vi "PicohrdlStreamingRun.vi"(5 "noOfChannels":i16=2, 7 "conversionTime":i16(ring) items=["60 ms", "100 ms", "180 ms", "340 ms", "660 ms"], 8 "error in (no error)":errorcluster, 9 "method":i16=2, 10 "nValues":i32=20, 11 "Handle in":i16) -> (0 "error out":errorcluster, 2 "sampleInterval_ms":i32, 3 "Handle out":i16)   [LabVIEW 2010]
doc: "Calls HRDLSetInterval() and HRDLRun() to setup sample interval and start streaming of data"
uses:
  PicoHRDL.dll
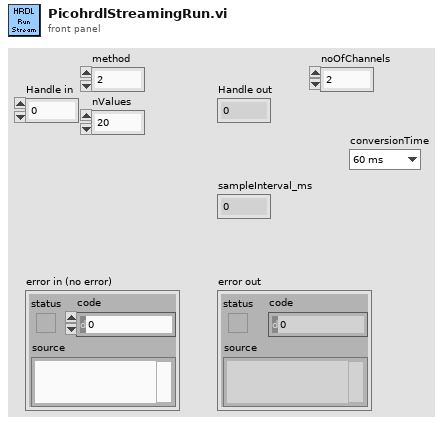
[diagram p1: front panel]
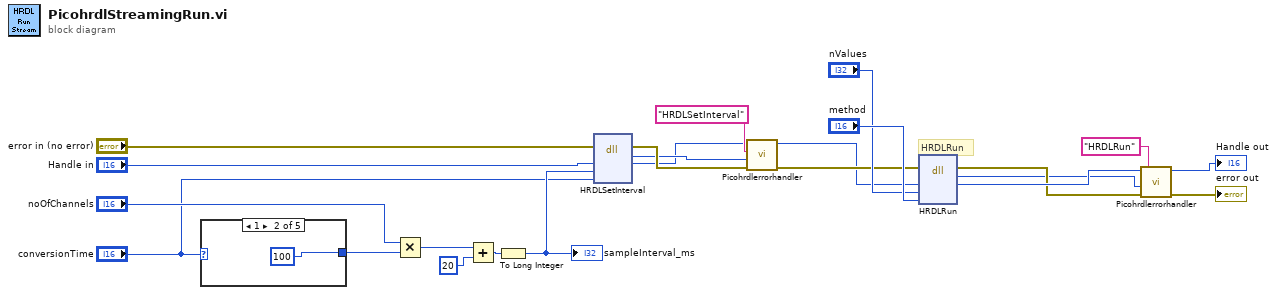
[diagram p0: block diagram]
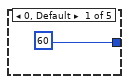
[diagram p2: hidden frame]
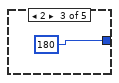
[diagram p3: hidden frame]
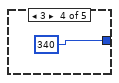
[diagram p4: hidden frame]
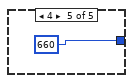
[diagram p5: hidden frame]
diagram:
  # "HRDLRun"
  n1 = case shown="1" "conversionTime" {
    tunnel: [60 ("32bit integer") 100 ("32bit integer") 180 ("32bit integer") 340 ("32bit integer") 660 ("32bit integer")] -> w18
    frame 0, Default {
    }
    frame 1 {
    }
    frame 2 {
    }
    frame 3 {
    }
    frame 4 {
    }
  }
  n2 = Multiply(x="noOfChannels", y=w18) -> (x*y=w23:i32)
  n3 = Add(x=w23, y=20) -> (x+y=w22:i32)
  n4 = To Long Integer(number=w22) -> (32bit integer=w17:i32)
  "sampleInterval_ms" <- w17
  n5 = dll-call lib="PicoHRDL.dll" fn="HRDLSetInterval"(error in="error in (no error)", "handle"="Handle in", "sampleInterval_ms"=w17, "conversionTime"="conversionTime") -> (error out=w3:errorcluster, "return type"=w2:i16, "handle"=w1:i16)  [unwired: 4 in, 1 out]
  n6 = call "Picohrdlerrorhandler.vi"("Handle in"=w1, "API function"="HRDLSetInterval", "Return"=w2, "error in (no error)"=w3) -> ("Handle out"=w4:i16, "error out"=w5:errorcluster)  [unwired: 5 in]
  n7 = dll-call lib="PicoHRDL.dll" fn="HRDLRun"(error in=w5, "handle"=w4, "nValues"="nValues", "method"="method") -> (error out=w7:errorcluster, "return type"=w6:i16, "handle"=w8:i16)  [unwired: 4 in, 1 out]
  n8 = call "Picohrdlerrorhandler.vi"("Handle in"=w8, "API function"="HRDLRun", "Return"=w6, "error in (no error)"=w7) -> ("Handle out"=→"Handle out":i16, "error out"=→"error out":errorcluster)  [unwired: 5 in]
